vi "Read output range.vi"(8 "error in (no error)":errorcluster, 11 "PID Loop in":refnum<class "PID Loop.lvclass">) -> (0 "error out":errorcluster, 2 "output range":T1={"output high"=100.0, "output low"=-100.0} {"output low" format="%.2f"; "output high" format="%.2f"}, 3 "PID Loop out":refnum<class "PID Loop.lvclass">)   [LabVIEW 2014, in "PID Loop.lvclass"]
uses:
  PID Loop.lvclass
  PID Range.ctl
  PID Loop.lvclass/PID Loop.ctl
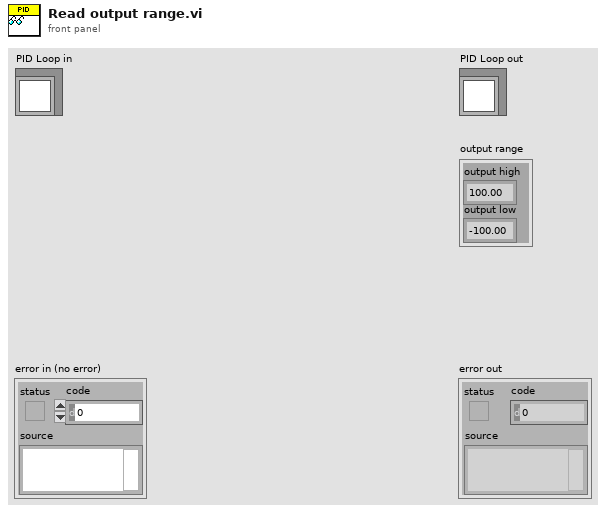
[diagram p1: front panel]
types:
  T1 = typedef "PID Loop.lvclass/PID Range.ctl" = cluster{"output high":dbl, "output low":dbl}
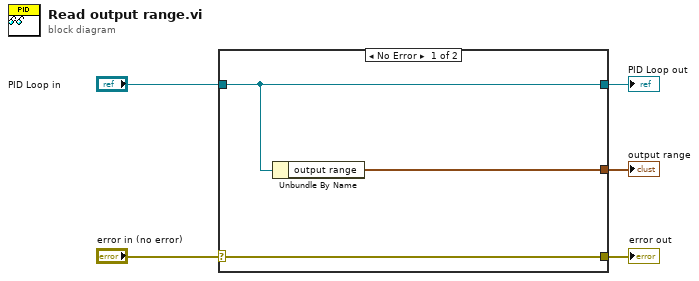
[diagram p0: block diagram]
diagram:
  n1 = case shown="No Error" "error in (no error)" {
    selector: "error in (no error)" -> [w8 w9]
    tunnel: [w8 w9] -> w4
    tunnel: [w7 w10] -> w2
    tunnel: "PID Loop in" -> [w7 w10]
    tunnel: [w6 _] -> w1
    frame No Error {
      n2 = Unbundle By Name(w7) -> ("output range"=w6:T1)
    }
    frame Error {
    }
  }
  "error out" <- w4
  "PID Loop out" <- w2
  "output range" <- w1
